vi "Initialize All SLM.vi"   [LabVIEW 2014]
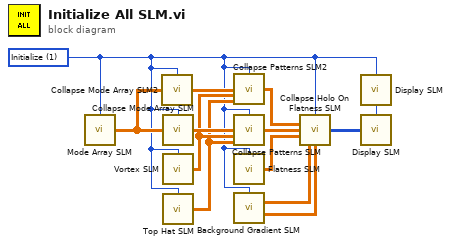
[diagram p0: block diagram]
diagram:
  w2 = u16 1 items=["Read", "Initialize"] ("Action")
  n1 = call "Mode Array SLM.vi"("Action"=w2) -> ("mode array"=w8:dbl[][][])  [unwired: 14 in]
  n2 = call "Collapse Mode Array SLM2.vi"("Action"=w2, "mode array"=w8) -> ("collapsed mode array"=w7:dbl[][])  [unwired: 13 in]
  n3 = call "Collapse Mode Array SLM.vi"("Action"=w2, "mode array"=w8) -> ("collapsed mode array"=w12:dbl[][])  [unwired: 13 in]
  n4 = call "Vortex SLM.vi"("Action"=w2) -> ("Vortex"=w6:dbl[][])  [unwired: 14 in]
  n5 = call "Top Hat SLM.vi"("Action"=w2) -> ("Top hat"=w5:dbl[][])  [unwired: 14 in]
  n6 = call "Collapse Patterns SLM2.vi"("Action"=w2, "collapsed mode array"=w7, "Vortex"=w6, "Top hat"=w5) -> ("collapsed patterns"=w4:dbl[][])  [unwired: 11 in]
  n7 = call "Collapse Patterns SLM.vi"("Action"=w2, "collapsed mode array"=w12, "Vortex"=w6, "Top hat"=w5) -> ("collapsed patterns"=w11:dbl[][])  [unwired: 11 in]
  n8 = call "Flatness SLM.vi"("Action"=w2) -> ("flatness"=w10:dbl[][])  [unwired: 14 in]
  n9 = call "Background Gradient SLM.vi"("Action"=w2) -> ("gradient"=w3:dbl[][], "holo mask"=w1:dbl[][])  [unwired: 13 in]
  n10 = call "Collapse Holo On Flatness SLM.vi"("Action"=w2, "collapsed patterns 2"=w4, "collapsed patterns"=w11, "flatness"=w10, "gradient"=w3, "holo mask"=w1) -> ("displayed matrix"=w9:u8[][])  [unwired: 9 in]
  n11 = call "Display SLM.vi"("Action"=w2) -> ("Read action"=w13:u16)  [unwired: 14 in]
  n12 = call "Display SLM.vi"("Action"=w13, "displayed matrix"=w9) -> ()  [unwired: 13 in, 1 out]
